vi "modify ROI when tracking.vi"(4 "Origin.Y":sgl, 6 "Origin.X":sgl, 8 "error in (no error)":errorcluster caption="错误输入（无错误）", 9 "new x y":cluster{"X":sgl, "Y":sgl}, 10 "ROI size num":i32[](array[numeric]), 11 "ROI Descriptor":T1 {"Contours"."Type" items=["No Selection", "Point", "Line", "Rectangle", "Oval", "Polygon", "Freehand Region", "Annulus", "Unused2", "Unused3", "Broken Line", "Freehand Line", "Rotated Rectangle"]}) -> (0 "error out":errorcluster caption="错误输出", 3 "ROI Descriptor out":T1 {"Contours"."Type" items=["No Selection", "Point", "Line", "Rectangle", "Oval", "Polygon", "Freehand Region", "Annulus", "Unused2", "Unused3", "Broken Line", "Freehand Line", "Rotated Rectangle"]})   [LabVIEW 2017]
doc: "本VI的功能是计算出修正后的衍射环中心位置后，对ROI进行修正，使得ROI的框始终跟随球的运动而运动。\n基本原理就是通过transform ROI 来修改ROI的位置。\n由于是队列的处理，更新不排除有一定的延迟，但是只对显示有影响，不对测量有影响。"
uses:
  <vilib>/vision/NI_Vision_Development_Module.lvlib
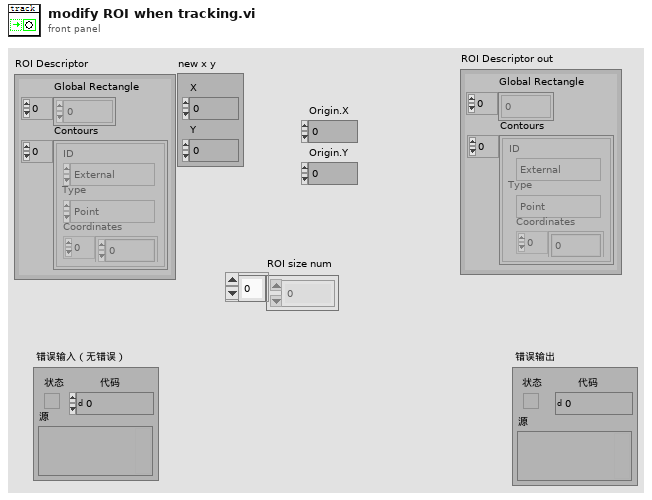
[diagram p1: front panel]
types:
  T1 = typedef "ROI Descriptor" = cluster{"Global Rectangle":i32[], "Contours":cluster{"ID":enum32{"External", "Internal"}, "Type":u32, "Coordinates":i32[]}[]}
  T2 = cluster{"Origin":cluster{"X":sgl, "Y":sgl}, "Angle (deg)":sgl, "Axis Reference":u32}
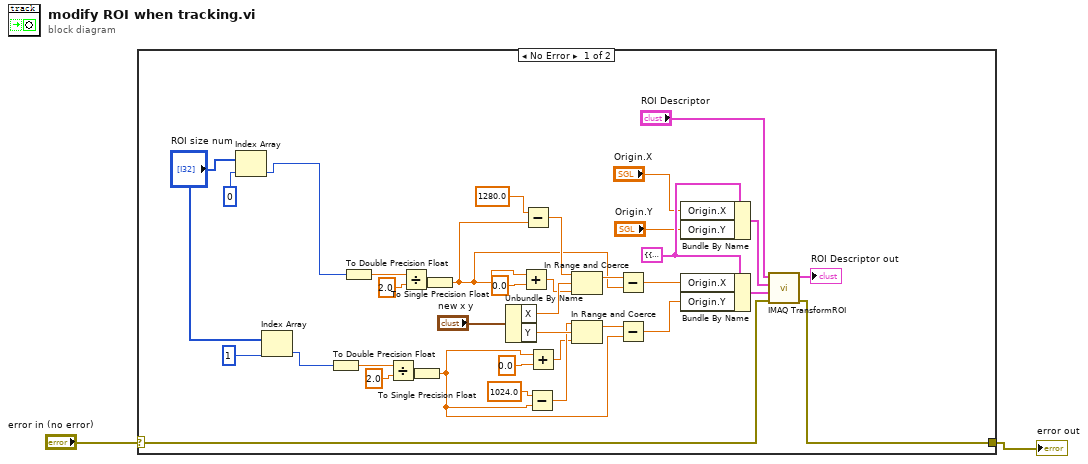
[diagram p0: block diagram]
diagram:
  n1 = case shown="No Error" "error in (no error)" {
    selector: "error in (no error)" -> [w39 w40]
    tunnel: [w38 w40] -> w1
    frame No Error {
      w33 = T2 {"Origin"={"X"=0.0, "Y"=0.0}, "Angle (deg)"=0.0, "Axis Reference"=0} ("Base Reference")
      n2 = Index Array(array="ROI size num", index=0 ("索引")) -> (element=w13:i32)
      n3 = Index Array(array="ROI size num", index=1 ("索引")) -> (element=w7:i32)
      n4 = To Double Precision Float(number=w7) -> (double precision float=w10:dbl)
      n5 = To Double Precision Float(number=w13) -> (double precision float=w25:dbl)
      n6 = Divide(x=w10, y=2.0) -> (x/y=w9:dbl)
      n7 = Divide(x=w25, y=2.0) -> (x/y=w26:dbl)
      n8 = To Single Precision Float(number=w9) -> (single precision float=w3:sgl)
      n9 = To Single Precision Float(number=w26) -> (single precision float=w4:sgl)
      n10 = Unbundle By Name("new x y") -> ("X"=w24:sgl, "Y"=w22:sgl)
      n11 = Add(x=w4, y=sgl 0.0 ("下限")) -> (x+y=w5:sgl)
      n12 = Subtract(x=sgl 1280.0 ("上限"), y=w4) -> (x-y=w19:sgl)
      n13 = Subtract(x=sgl 1024.0 ("上限"), y=w3) -> (x-y=w17:sgl)
      n14 = Add(x=w3, y=sgl 0.0 ("下限")) -> (x+y=w15:sgl)
      n15 = In Range and Coerce(upper limit=w19, x=w24, lower limit=w5) -> (coerced(x)=w23:sgl)  [unwired: 1 out]
      n16 = In Range and Coerce(upper limit=w17, x=w22, lower limit=w15) -> (coerced(x)=w21:sgl)  [unwired: 1 out]
      n17 = Subtract(x=w23, y=w4) -> (x-y=w29:sgl)
      n18 = Subtract(x=w21, y=w3) -> (x-y=w28:sgl)
      n19 = Bundle By Name(cluster=w33, "Origin.X"="Origin.X", "Origin.Y"="Origin.Y") -> (w34:T2)
      n20 = Bundle By Name(cluster=w33, "Origin.X"=w29, "Origin.Y"=w28) -> (w36:T2)
      n21 = call "IMAQ TransformROI"("error in (no error)"=w39, "New Reference"=w36, "Base Reference"=w34, "ROI Descriptor"="ROI Descriptor") -> ("error out"=w38:errorcluster, "ROI Descriptor out"=→"ROI Descriptor out":T1)  [unwired: 6 in]
    }
    frame Error {
    }
  }
  "error out" <- w1
